vi "Resonance_CalculateSubset.vi"(8 "error in":errorcluster, 11 "FGEN Parameters":T1 {"Trigger Mode" items=["Single", "Continuous", "Stepped", "Burst"]}) -> (0 "error out":errorcluster, 1 "dF":dbl, 2 "Length":i32, 3 "Index":i32, 4 "Start Offset":dbl)   [LabVIEW 2023, in "Resonance.lvlib"]
doc: "Calculates the subset parameters of the FFT considering the sample rate, the Start Frequency/Stop Frequency of the Chirp waveform and the number of samples"
uses:
  Resonance.lvlib
  ResourceHandling/TypeDefs/RH_FGEN_Parameters.ctl
  <instrlib>/niFgen/niFgen.llb/niFgen Trigger Mode.ctl
  ResourceHandling/ResourceHandling.lvlib
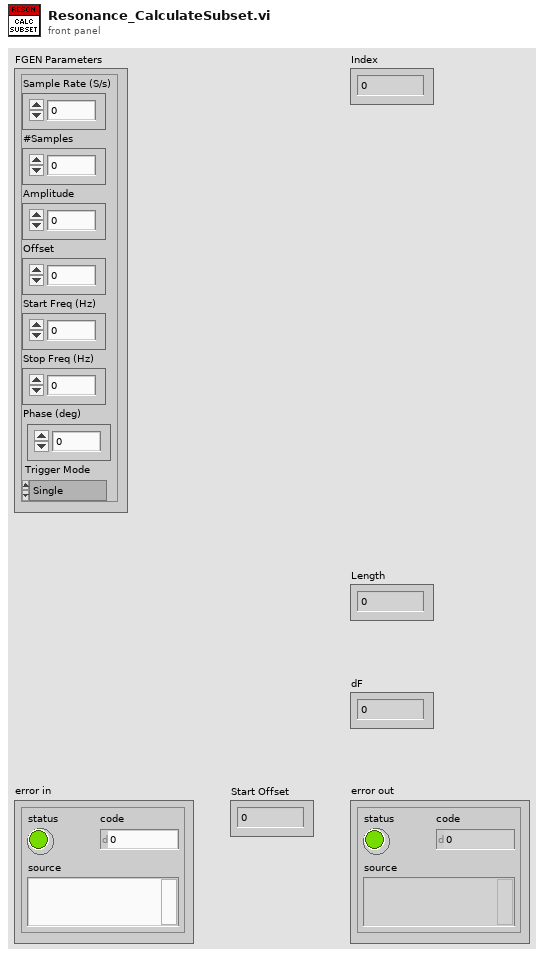
[diagram p1: front panel]
types:
  T1 = typedef "ResourceHandling.lvlib/RH_FGEN_Parameters.ctl" = cluster{"Sample Rate (S/s)":dbl, "#Samples":i32, "Amplitude":dbl, "Offset":dbl, "Start Freq (Hz)":dbl, "Stop Freq (Hz)":dbl, "Phase (deg)":dbl, "Trigger Mode":T2}
  T2 = typedef "niFgen Trigger Mode.ctl" = i32
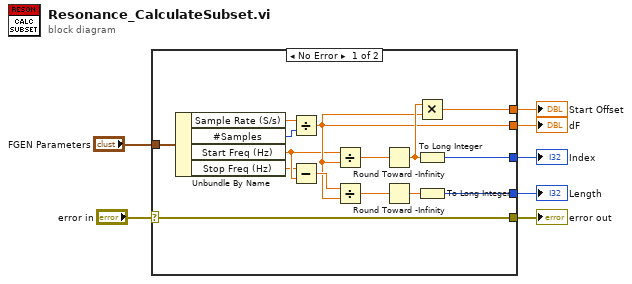
[diagram p0: block diagram]
diagram:
  n1 = case shown="No Error" "error in" {
    selector: "error in" -> [w8 w23]
    tunnel: "FGEN Parameters" -> [w22 _]
    tunnel: [w16 _] -> w6
    tunnel: [w11 _] -> w5
    tunnel: [w10 _] -> w4
    tunnel: [w9 _] -> w3
    tunnel: [w8 w23] -> w1
    frame No Error {
      n2 = Unbundle By Name(w22) -> ("Sample Rate (S/s)"=w12:dbl, "#Samples"=w15:i32, "Start Freq (Hz)"=w14:dbl, "Stop Freq (Hz)"=w13:dbl)
      n3 = Divide(x=w12, y=w15) -> (x/y=w16:dbl)
      n4 = Subtract(x=w13, y=w14) -> (x-y=w21:dbl)
      n5 = Divide(x=w14, y=w16) -> (x/y=w20:dbl)
      n6 = Divide(x=w21, y=w16) -> (x/y=w19:dbl)
      n7 = Round Toward -Infinity(1:w20) -> (0:w17:dbl)
      n8 = Round Toward -Infinity(1:w19) -> (0:w18:dbl)
      n9 = Multiply(x=w17, y=w16) -> (x*y=w10:dbl)
      n10 = To Long Integer(number=w17) -> (32bit integer=w11:i32)
      n11 = To Long Integer(number=w18) -> (32bit integer=w9:i32)
    }
    frame Error {
    }
  }
  "Index" <- w5
  "Start Offset" <- w4
  "Length" <- w3
  "dF" <- w6
  "error out" <- w1
